vi "set_params.vi"(8 "error in (no error)":errorcluster, 11 "stresing in":refnum<class "stresing.lvclass">) -> (0 "error out":errorcluster, 3 "stresing out":refnum<class "stresing.lvclass">)   [LabVIEW 2019, in "stresing.lvlib" / "stresing.lvclass"]
uses:
  stresing.lvclass
  stresing.lvclass/stresing.ctl
panel:
  in  "driver path":path
  in  "OK Button":bool
  in  "number of blocks":u32
  in  "number of spectra":u32
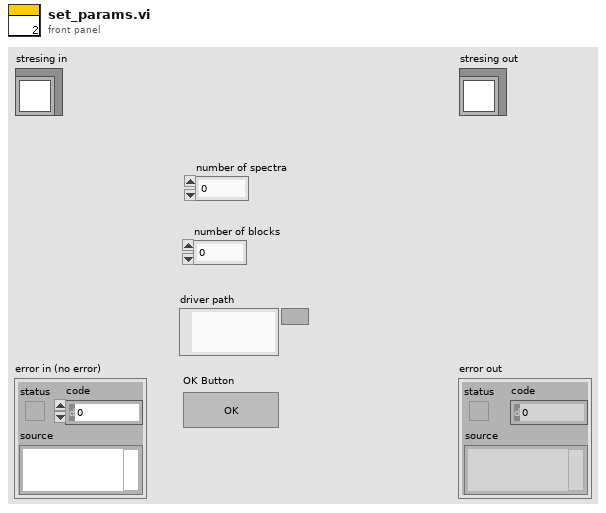
[diagram p1: front panel]
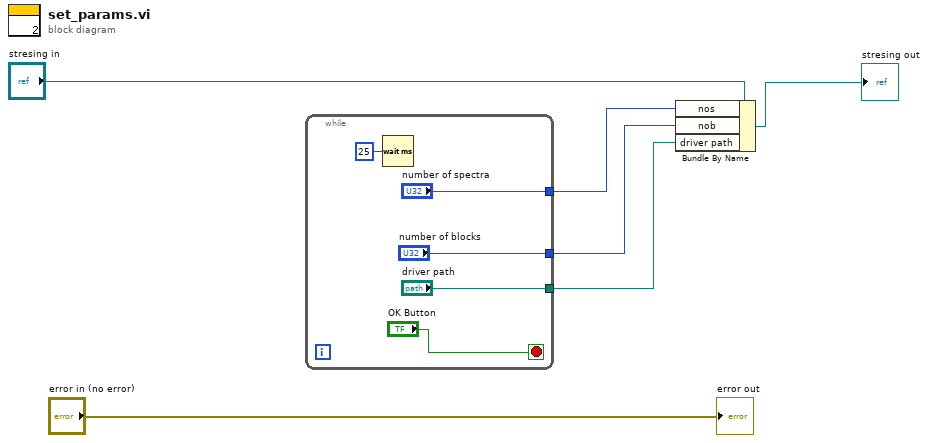
[diagram p0: block diagram]
diagram:
  n1 = while {
    tunnel: ["number of spectra"] -> w4
    tunnel: ["number of blocks"] -> w3
    tunnel: ["driver path"] -> w1
    stop <- "OK Button" stop-if-true
    n2 = Wait (ms)(milliseconds to wait=u32 25) -> ()  [unwired: 1 out]
  }
  n3 = Bundle By Name(cluster="stresing in", "nos"=w4, "nob"=w3, "driver path"=w1) -> (→"stresing out":refnum<class "stresing.lvclass">)
  "error out" <- "error in (no error)"
